vi "Configure BinWidth.vi"(8 "error in (no error)":errorcluster, 10 "BinWidth":dbl[unit], 11 "CS++MCS in":refnum<class "CS++MCS.lvclass">) -> (0 "error out":errorcluster, 3 "CS++MCS out":refnum<class "CS++MCS.lvclass">)   [LabVIEW 2015, in "CS++MCS.lvlib" / "CS++MCS.lvclass"]
doc: "This VI configures the Bin Width of the recorded spectrum.\nNote that depending on the used device the actual set value will be rounded."
uses:
  CS++MCS.lvclass
  CSPP_Core/Classes/CS++ProcessVariables/ProcessVariable/PV.lvclass
  CSPP_Core/Classes/CS++ProcessVariables/ProcessVariable/PV.lvclass/PV.ctl
  CS++MCS.lvclass/CS++MCS.ctl
  CSPP_Core/Classes/CS++ProcessVariables/ProcessVariable/Write Data.vi
  CSPP_Core/Classes/CS++ProcessVariables/ProcessVariable/Write Timestamp.vi
  CSPP_Core/Classes/CS++ProcessVariables/ProcessVariable/Write Quality.vi
  CSPP_Core/Classes/CS++ProcessVariables/ProcessVariable/Write status.vi
  CSPP_Core/Classes/CS++ProcessVariables/PVConnection/PVConnection.lvclass
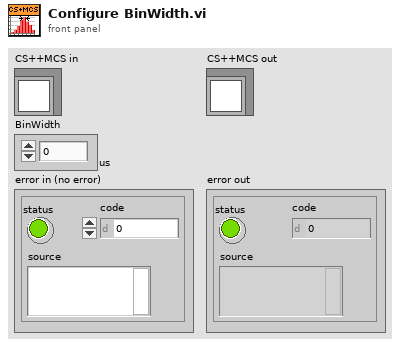
[diagram p1: front panel]
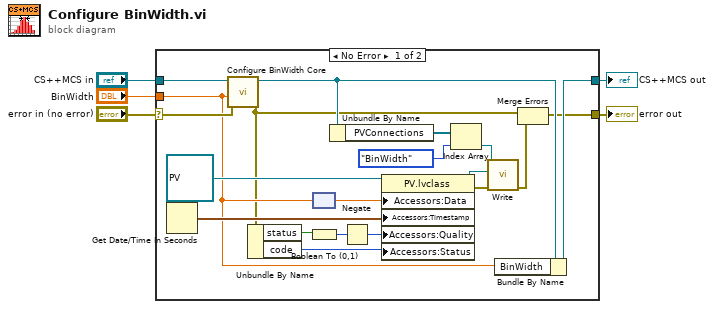
[diagram p0: block diagram]
diagram:
  n1 = case shown="No Error" "error in (no error)" {
    selector: "error in (no error)" -> [w24 w27]
    tunnel: [w7 w27] -> w4
    tunnel: [w10 w26] -> w2
    tunnel: "CS++MCS in" -> [w25 w26]
    tunnel: "BinWidth" -> [w9 _]
    frame No Error {
      n2 = Get Date/Time In Seconds() -> (seconds since 1Jan1904=w14:timestamp)
      n3 = call-dynamic "Configure BinWidth Core.vi"("error in (no error)"=w24, "BinWidth"=w9, "CS++MCS in"=w25) -> ("error out"=w8:errorcluster, "CS++MCS out"=w11:refnum<class "CS++MCS.lvclass">)  [unwired: 7 in]
      n4 = Unbundle By Name(w8) -> ("status"=w18:bool, "code"=w20:i32)
      n5 = Boolean To (0,1)(Boolean=w18) -> (0, 1=w19:i16)
      n6 = node(w9) -> (w13:dbl)
      n7 = Unbundle By Name(w11) -> ("PVConnections"=w23:refnum<class "PVConnection.lvclass">[])
      n8 = Negate(x=w19) -> (-x=w21:i16)
      n9 = property class="PV.lvclass"(reference=refnum<class "PV.lvclass"> refnum ("PV"), "Accessors:Data"=w13, "Accessors:Timestamp"=w14, "Accessors:Quality"=w21, "Accessors:Status"=w20) -> (reference out=w17:refnum<class "PV.lvclass">, error out=w16:errorcluster)  [unwired: 1 in]
      n10 = Index Array(array=w23, index=enum16{"BinWidth"}."BinWidth" ("PV-Enum")) -> (element=w12:refnum<class "PVConnection.lvclass">)
      n11 = call "Write.vi"("error in (no error)"=w16, "PV"=w17, "PVConnection in"=w12) -> ("error out"=w6:errorcluster)  [unwired: 7 in, 1 out]
      n12 = Bundle By Name(cluster=w11, "BinWidth"=w9) -> (w10:refnum<class "CS++MCS.lvclass">)
      n13 = Merge Errors(w8, w6) -> (w7:errorcluster)
    }
    frame Error {
    }
  }
  "error out" <- w4
  "CS++MCS out" <- w2
